vi "tsdb_unload_can_dbs_win32.vi"(8 "错误输入（无错误）":errorcluster) -> (0 "错误输出":errorcluster, 3 "tsdb_unload_can_dbs":i32)   [LabVIEW 2016]
uses:
  TSMaster.dll
panel:
  # "卸载所有的dbc,并释放dbc的内存"
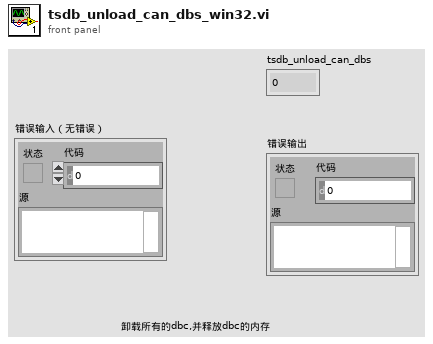
[diagram p1: front panel]
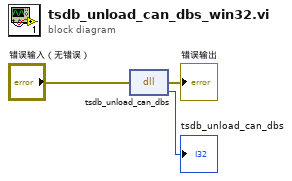
[diagram p0: block diagram]
diagram:
  n1 = dll-call lib="C:/Users/Eric/Desktop/LabVIEW/TSMasterAPI/Win32/CANopen_TS_2015/TSMaster.dll" fn="tsdb_unload_can_dbs"(error in="错误输入（无错误）") -> (error out=→"错误输出":errorcluster, "tsdb_unload_can_dbs"=→"tsdb_unload_can_dbs":i32)  [unwired: 2 in, 1 out]
